vi "gaussmeter_config_DC.vi"(8 "error in (no error)":errorcluster, 11 "VISA Refnum in":refnum<visa-resource-name>) -> (0 "error out":errorcluster, 3 "VISA Refnum out":refnum<visa-resource-name>)   [LabVIEW 2017]
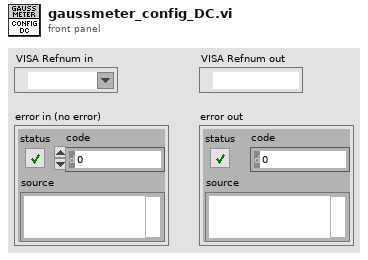
[diagram p1: front panel]
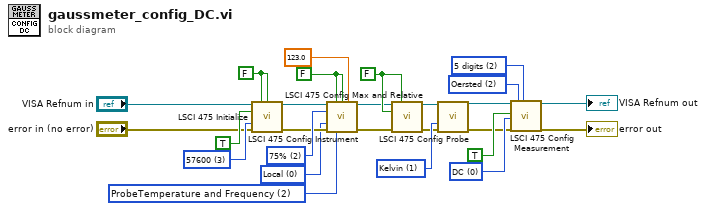
[diagram p0: block diagram]
diagram:
  w21 = u16 2 items=["Blank", "Field", "ProbeTemperature and Frequency", "Relative Setpoint", "Field Control Setpoint", "Alarm Sort Message"] ("Display Line 2 (0: Blank)")
  w20 = u16 2 items=["25%", "50%", "75%", "100%"] ("Display Brightness (0: 75%)")
  w17 = u16 2 items=["3 digits", "4 digits", "5 digits"] ("DC Resolution (0: 3 digits)")
  w16 = u16 2 items=["Gauss", "Tesla", "Oersted", "Amp/meter"] ("Field Units (0: Gauss)")
  w15 = u16 0 items=["DC", "RMS", "Peak"] ("Measurement Mode (0: DC)")
  w11 = u16 1 items=["Celsius", "Kelvin"] ("Temperature Units (0: Celsius)")
  w26 = FALSE ("Relative Mode (F: Off)")
  w6 = u16 0 items=["Local", "Remote", "Remote with Local Lockout"] ("Remote Interface Mode (0: Local)")
  w25 = FALSE ("Keyboard Lock (F: Unlocked)")
  w4 = 3 items=["9600", "19200", "38400", "57600"] ("Baud Rate (0: 9600)")
  w24 = FALSE ("Reset Defaults (F:Dont Reset)")
  n1 = call <instrlib>:"LSCI 475 Initialize.vi"("VISA Resource Name"="VISA Refnum in", "Reset (T: Reset)"=w24, "Reset Defaults (F:Dont Reset)"=w24, "ID Query (T: Check)"=TRUE, "Baud Rate (0: 9600)"=w4, "error in (no error)"="error in (no error)") -> ("VISA session"=w18:refnum<visa-resource-name>, "error out"=w19:errorcluster)  [unwired: 8 in]
  n2 = call <instrlib>:"LSCI 475 Config Instrument.vi"("VISA session"=w18, "Beep (F: Off)"=w25, "Keyboard Lock (F: Unlocked)"=w25, "Keyboard Lock Code (123)"=123.0, "Display Brightness (0: 75%)"=w20, "Remote Interface Mode (0: Local)"=w6, "error in (no error)"=w19, "Display Line 2 (0: Blank)"=w21) -> ("dup VISA session"=w7:refnum<visa-resource-name>, "error out"=w8:errorcluster)  [unwired: 6 in]
  n3 = call <instrlib>:"LSCI 475 Config Max and Relative.vi"("VISA session"=w7, "Relative Mode (F: Off)"=w26, "Max Hold (F: Off)"=w26, "error in (no error)"=w8) -> ("dup VISA session"=w9:refnum<visa-resource-name>, "error out"=w10:errorcluster)  [unwired: 10 in]
  n4 = call <instrlib>:"LSCI 475 Config Probe.vi"("VISA session"=w9, "Temperature Units (0: Celsius)"=w11, "error in (no error)"=w10) -> ("dup VISA session"=w12:refnum<visa-resource-name>, "error out"=w13:errorcluster)  [unwired: 11 in]
  n5 = call <instrlib>:"LSCI 475 Config Measurement.vi"("VISA session"=w12, "Auto Range (F: Off)"=TRUE, "Measurement Mode (0: DC)"=w15, "error in (no error)"=w13, "Field Units (0: Gauss)"=w16, "DC Resolution (0: 3 digits)"=w17) -> ("dup VISA session"=→"VISA Refnum out":refnum<visa-resource-name>, "error out"=→"error out":errorcluster)  [unwired: 12 in]
